vi "PulseGenerator.vi"(11 "x":i32) -> (3 "Boolean":bool)   [LabVIEW 2019]
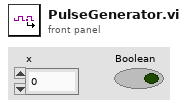
[diagram p1: front panel]
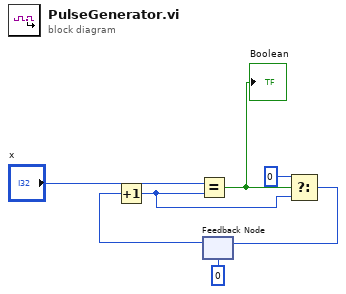
[diagram p0: block diagram]
diagram:
  n1 = feedback #1(0) -> (w6:i32)
  n2 = Increment(x=w6) -> (x+1=w3:i32)
  n3 = Equal?(x="x", y=w3) -> (x = y?=w1:bool)
  "Boolean" <- w1
  n4 = Select(t=0 ("x"), s=w1, f=w3) -> (s? t:f=w2:i32)
  n5 = feedback-in #1(w2) -> ()
